vi "Charger_Monitor Loop.vi"(6 "Stop Refnum":refnum<vi>, 7 "Status Refnum":T2, 8 "error in":errorcluster, 9 "semaphore":T1) -> (0 "error out":errorcluster, 1 "semaphore out":T1)   [LabVIEW 2020]
uses:
  Charger_Status Refnum.ctl
  Drivers/Charger Test Set/Charger_Input Control.ctl
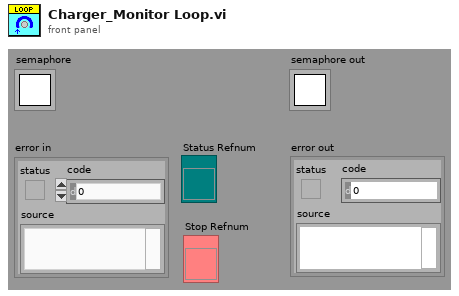
[diagram p1: front panel]
types:
  T1 = typedef "Semaphore RefNum" = refnum<k1>
  T2 = typedef "Charger_Status Refnum.ctl" = refnum<vi>
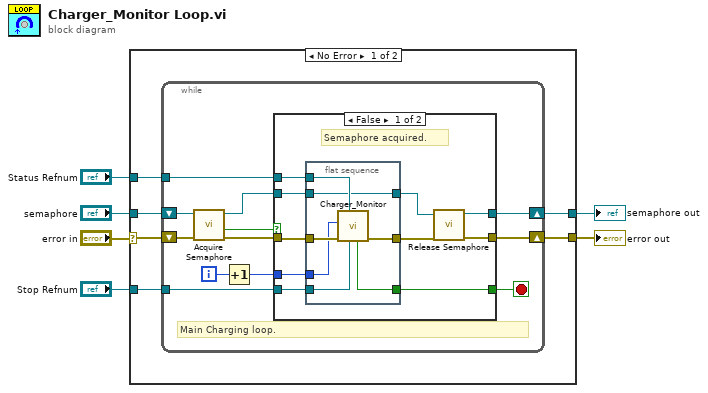
[diagram p0: block diagram]
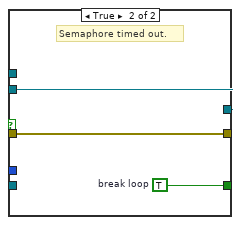
[diagram p2: hidden frame]
diagram:
  n1 = case shown="No Error" "error in" {
    selector: "error in" -> [w7 w46]
    tunnel: "semaphore" -> [w12 w45]
    tunnel: "Stop Refnum" -> [w11 _]
    tunnel: [w10 w46] -> w4
    tunnel: [w9 w45] -> w3
    tunnel: "Status Refnum" -> [w8 _]
    frame No Error {
      n2 = while {
        shift-right: [w16] -> w10
        shift-left: w7 -> [w20]
        shift-right: [w21] -> w9
        shift-left: w12 -> [w24]
        tunnel: w11 -> [w19]
        tunnel: w8 -> [w18]
        i -> [w15]
        stop <- w14 stop-if-true
        # "Main Charging loop."
        n3 = call <vilib>:"Acquire Semaphore.vi"("error in (no error)"=w20, "semaphore"=w24) -> ("error out"=w17:errorcluster, "timed out"=w22:bool, "semaphore out"=w23:T1)  [unwired: 3 in]
        n4 = Increment(x=w15) -> (x+1=w13:i32)
        n5 = case shown="False" w22 {
          tunnel: w17 -> [w30 w43]
          tunnel: [w33 w43] -> w16
          tunnel: w23 -> [w26 w44]
          tunnel: [w34 w44] -> w21
          tunnel: w19 -> [w31 _]
          tunnel: w18 -> [w32 _]
          tunnel: w13 -> [w29 _]
          tunnel: [w27 w42] -> w14
          frame False {
            # "Semaphore acquired."
            n6 = flat-sequence {
              tunnel: w32 -> [w41]
              tunnel: w31 -> [w40]
              tunnel: w30 -> [w39]
              tunnel: w29 -> [w38]
              tunnel: [w37] -> w28
              tunnel: [w36] -> w27
              tunnel: w26 -> [w35]
              tunnel: [w35] -> w25
              frame #0 {
                n7 = call "Charger_Monitor.vi"("Stop Refnum"=w40, "Status Refnum"=w41, "error in"=w39, "Index"=w38) -> ("error out"=w37:errorcluster, "done"=w36:bool)  [unwired: 6 in]
              }
            }
            n8 = call <vilib>:"Release Semaphore.vi"("error in (no error)"=w28, "semaphore"=w25) -> ("error out"=w33:errorcluster, "semaphore out"=w34:T1)  [unwired: 4 in]
          }
          frame True {
            w42 = TRUE  # break loop
            # "Semaphore timed out."
          }
        }
      }
    }
    frame Error {
    }
  }
  "error out" <- w4
  "semaphore out" <- w3
